vi "Validate Inputs.vi"(8 "error in":errorcluster, 11 "CDPW_MetaDataObj":refnum<class "NIVS_CDEW_MetaDataObj.lvclass">) -> (0 "error out":errorcluster, 3 "CDPW_MetaDataObj":refnum<class "NIVS_CDEW_MetaDataObj.lvclass">)   [LabVIEW 2026, in "NIVS_CDEW_MetaDataObj.lvclass"]
uses:
  NIVS_CDEW_MetaDataObj.lvclass
  NIVS_CDEW_MetaDataObj.lvclass/NIVS_CDEW_MetaDataObj.ctl
  Types/Errors.ctl
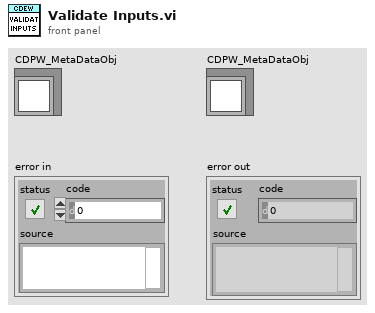
[diagram p1: front panel]
types:
  T1 = enum16{"Validate XML File", "Folder Path for Edit", "CD Root Path"}[]
  T2 = typedef "NIVS_CDEW_MetaDataObj.lvclass/Errors.ctl" = i32
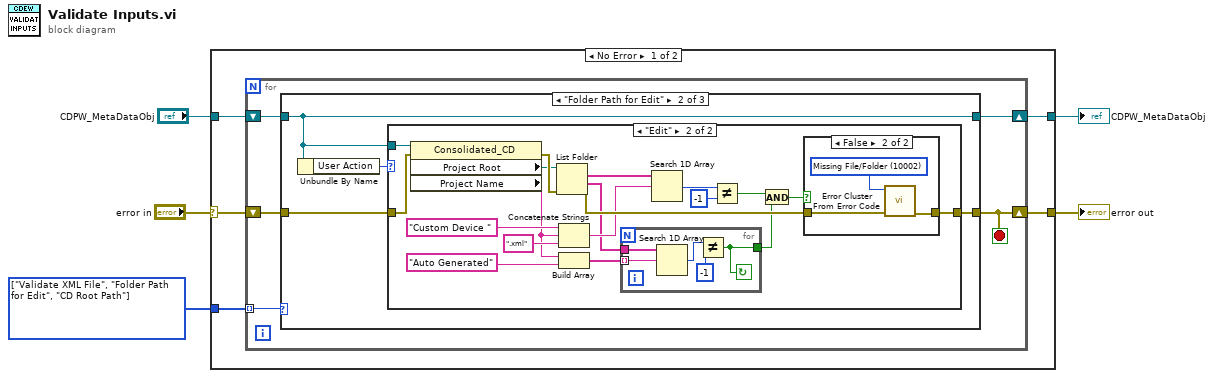
[diagram p0: block diagram]
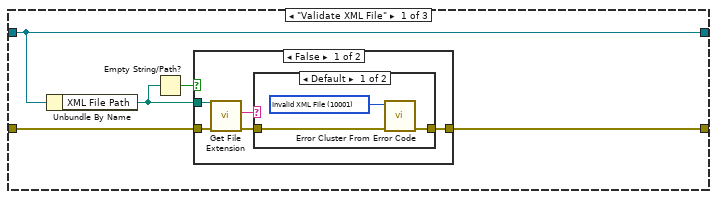
[diagram p2: hidden frame]
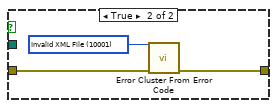
[diagram p4: hidden frame]
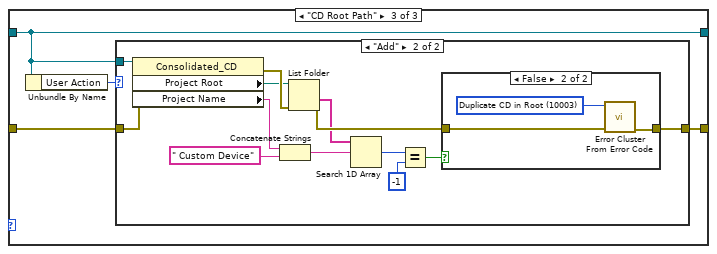
[diagram p7: hidden frame]
diagram:
  w1 = T1 [enum."Validate XML File", enum."Folder Path for Edit", enum."CD Root Path"] items=["Validate XML File", "Folder Path for Edit", "CD Root Path"]
  n1 = case shown="No Error" "error in" {
    selector: "error in" -> [w10 w89]
    tunnel: [w9 w89] -> w4
    tunnel: "CDPW_MetaDataObj" -> [w8 w88]
    tunnel: [w7 w88] -> w2
    tunnel: w1 -> [w6 _]
    frame No Error {
      n2 = for {
        shift-right: [w14] -> w9
        shift-left: w10 -> [w15]
        shift-right: [w12] -> w7
        shift-left: w8 -> [w13]
        tunnel: w6 -> [w11] mode=indexing
        stop <- w14 stop-if-true
        n3 = case shown="\"Folder Path for Edit\"" w11 {
          tunnel: w15 -> [w20 w36 w69]
          tunnel: w13 -> [w16 w33 w66]
          tunnel: [w19 w35 w68] -> w14
          tunnel: [w16 w33 w66] -> w12
          frame "Validate XML File" {
            n4 = Unbundle By Name(w16) -> ("XML File Path"=w17:path)
            n5 = Empty String/Path?(string/path=w17) -> (empty?=w18:bool)
            n6 = case shown="False" w18 {
              tunnel: w20 -> [w25 w31]
              tunnel: [w24 w32] -> w19
              tunnel: w17 -> [w22 _]
              frame False {
                n7 = call <vilib>:"Get File Extension.vi"("error in (no error)"=w25, "file"=w22) -> ("error out"=w23:errorcluster, "lowercase file extension"=w21:string)  [unwired: 5 in, 3 out]
                n8 = case shown="Default" w21 {
                  tunnel: [w28 w29] -> w24
                  tunnel: w23 -> [w27 w29]
                  frame Default {
                    w26 = T2 10001 items=["Invalid XML File"=10001, "Missing File/Folder"=10002, "Duplicate CD in Root"=10003] ("Errors")
                    n9 = call <vilib>:"Error Cluster From Error Code.vi"("error in (no error)"=w27, "error code (0)"=w26) -> ("error out"=w28:errorcluster)  [unwired: 7 in]
                  }
                  frame "xml" {
                  }
                }
              }
              frame True {
                w30 = T2 10001 items=["Invalid XML File"=10001, "Missing File/Folder"=10002, "Duplicate CD in Root"=10003] ("Errors")
                n10 = call <vilib>:"Error Cluster From Error Code.vi"("error in (no error)"=w31, "error code (0)"=w30) -> ("error out"=w32:errorcluster)  [unwired: 7 in]
              }
            }
          }
          frame "Folder Path for Edit" {
            n11 = Unbundle By Name(w33) -> ("User Action"=w34:enum16{"Add", "Edit"})
            n12 = case shown="\"Edit\"" w34 {
              tunnel: w33 -> [_ w52]
              tunnel: w36 -> [w37 w56]
              tunnel: [w37 w54] -> w35
              frame Default {
              }
              frame "Edit" {
                n13 = property class="Consolidated_CD"(reference=w52, error in=w56) -> (error out=w55:errorcluster, "Project Root"=w51:path, "Project Name"=w41:string)  [unwired: 1 out]
                n14 = List Folder(path=w51, error in=w55) -> (filenames=w50:string[], folder names=w43:string[], error out=w53:errorcluster)  [unwired: 2 in, 1 out]
                n15 = Concatenate Strings("Custom Device " ("element"), w41, ".xml" ("string")) -> (w47:string)
                n16 = Build Array(w41, "Auto Generated") -> (w42:string[])
                n17 = for {
                  tunnel: w43 -> [w61]
                  tunnel: w42 -> [w60] mode=indexing
                  tunnel: [w57] -> w38
                  stop <- w57 continue-if-true
                  n18 = Search 1D Array(1D array=w61, element=w60) -> (index of element=w59:i32)  [unwired: 1 in]
                  n19 = Not Equal?(x=w59, y=-1) -> (x != y?=w57:bool)
                }
                n20 = Search 1D Array(1D array=w50, element=w47) -> (index of element=w46:i32)  [unwired: 1 in]
                n21 = Not Equal?(x=w46, y=-1) -> (x != y?=w39:bool)
                n22 = And(x=w39, y=w38) -> (x .and. y?=w44:bool)
                n23 = case shown="False" w44 {
                  tunnel: [w62 w64] -> w54
                  tunnel: w53 -> [w62 w65]
                  frame True {
                  }
                  frame False {
                    w63 = T2 10002 items=["Invalid XML File"=10001, "Missing File/Folder"=10002, "Duplicate CD in Root"=10003] ("Errors")
                    n24 = call <vilib>:"Error Cluster From Error Code.vi"("error in (no error)"=w65, "error code (0)"=w63) -> ("error out"=w64:errorcluster)  [unwired: 7 in]
                  }
                }
              }
            }
          }
          frame "CD Root Path" {
            n25 = Unbundle By Name(w66) -> ("User Action"=w67:enum16{"Add", "Edit"})
            n26 = case shown="\"Add\"" w67 {
              tunnel: w66 -> [_ w79]
              tunnel: w69 -> [w70 w83]
              tunnel: [w70 w81] -> w68
              frame Default {
              }
              frame "Add" {
                n27 = property class="Consolidated_CD"(reference=w79, error in=w83) -> (error out=w82:errorcluster, "Project Root"=w78:path, "Project Name"=w76:string)  [unwired: 1 out]
                n28 = Concatenate Strings(w76, " Custom Device" ("string")) -> (w72:string)
                n29 = List Folder(path=w78, error in=w82) -> (folder names=w77:string[], error out=w80:errorcluster)  [unwired: 2 in, 2 out]
                n30 = Search 1D Array(1D array=w77, element=w72) -> (index of element=w75:i32)  [unwired: 1 in]
                n31 = Equal?(x=w75, y=-1) -> (x = y?=w73:bool)
                n32 = case shown="False" w73 {
                  tunnel: [w84 w86] -> w81
                  tunnel: w80 -> [w84 w87]
                  frame True {
                  }
                  frame False {
                    w85 = T2 10003 items=["Invalid XML File"=10001, "Missing File/Folder"=10002, "Duplicate CD in Root"=10003] ("Errors")
                    n33 = call <vilib>:"Error Cluster From Error Code.vi"("error in (no error)"=w87, "error code (0)"=w85) -> ("error out"=w86:errorcluster)  [unwired: 7 in]
                  }
                }
              }
            }
          }
        }
      }
    }
    frame Error {
    }
  }
  "error out" <- w4
  "CDPW_MetaDataObj" <- w2
